vi "Single Calculate Limit Test.vi"(8 "error in":errorcluster, 9 "Source":i32(ring) items=["Input Channel 1", "Input Channel 2", "Input Channel 3", "Input Channel 4", "Calc Channel 1", "Calc Channel 2", "Calc Channel 3", "Calc Channel 4", "Ref Channel 1", "Ref Channel 2", "Ref Channel 3", "Ref Channel 4"], 10 "Calculation Channel":i32(ring) items=["Calc Channel 1", "Calc Channel 2", "Calc Channel 3", "Calc Channel 4"], 11 "Instrument Handle In":i32) -> (0 "error out":errorcluster, 3 "Instrument Handle Out":i32)   [LabVIEW 8.6, in "ZTScopeM.lvlib"]
doc: "Configure a calculation channel to perform a limit test."
uses:
  ZTScopeM.lvlib
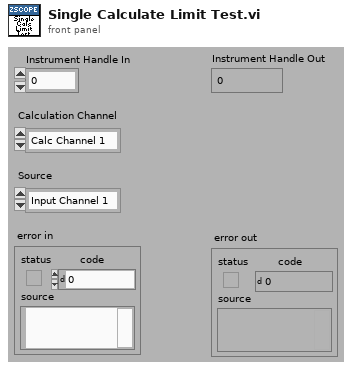
[diagram p1: front panel]
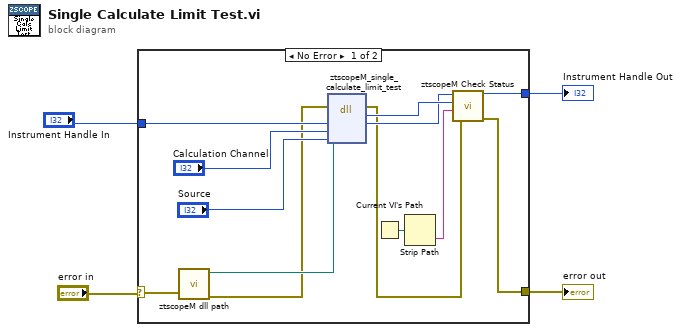
[diagram p0: block diagram]
diagram:
  n1 = case shown="No Error" "error in" {
    selector: "error in" -> [w9 w19]
    tunnel: [w12 w19] -> w3
    tunnel: [w13 w18] -> w2
    tunnel: "Instrument Handle In" -> [w7 w18]
    frame #0 {
      n2 = call "ztscopeM dll path.vi"("error in (no error)"=w9) -> ("error out"=w6:errorcluster, "<instrument>.dll path"=w8:path)  [unwired: 9 in]
      n3 = dll-call lib="C:/Program Files (x86)/National Instruments/LabVIEW 2013/instr.lib/ztscopem/ztscopeM.dll" fn="ztscopeM_single_calculate_limit_test"(path in=w8, error in=w6, "instrumentHandle"=w7, "calculationChannel"="Calculation Channel", "source"="Source") -> (error out=w5:errorcluster, w17:i32, "instrumentHandle"=w16:i32)  [unwired: 3 in, 1 out]
      n4 = Current VI's Path() -> (path=w15:path)
      n5 = Strip Path(path=w15) -> (name=w14:string)  [unwired: 1 out]
      n6 = call "ztscopeM Check Status.vi"("error in"=w5, "name of VI"=w14, "status (return code)"=w17, "instrument handle in"=w16) -> ("error out"=w12:errorcluster, "instrument handle out"=w13:i32)  [unwired: 2 out]
    }
    frame #1 {
    }
  }
  "Instrument Handle Out" <- w2
  "error out" <- w3
